vi "Simulate.vi"(8 "error in (no error)":errorcluster, 11 "Process Simulator in":refnum<class "Process Simulator.lvclass">) -> (0 "error out":errorcluster, 3 "Process Simulator out":refnum<class "Process Simulator.lvclass">)   [LabVIEW 2025, in "PID.lvlib" / "Process Simulator.lvclass"]
uses:
  Process Simulator.lvclass
  Process Simulator.lvclass/Process Simulator.ctl
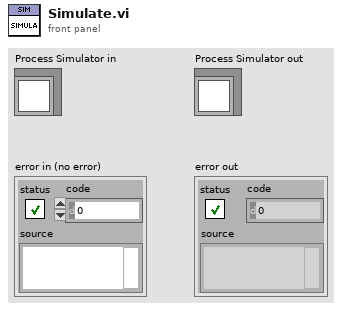
[diagram p1: front panel]
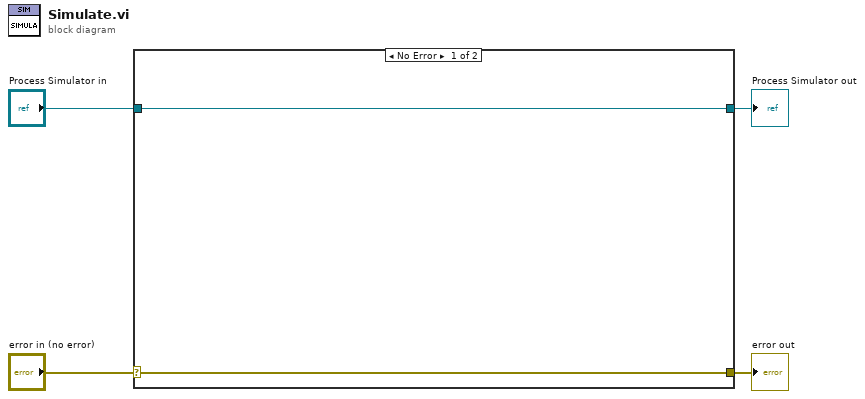
[diagram p0: block diagram]
diagram:
  n1 = case shown="No Error" "error in (no error)" {
    selector: "error in (no error)" -> [w5 w8]
    tunnel: [w5 w8] -> w3
    tunnel: [w6 w7] -> w1
    tunnel: "Process Simulator in" -> [w6 w7]
    frame No Error {
    }
    frame Error {
    }
  }
  "error out" <- w3
  "Process Simulator out" <- w1
